vi "Get Parameters And Check Data Types.vi"(8 "error in":errorcluster, 11 "variant":variant) -> (0 "error out":errorcluster, 2 "parameters with invalid type":string[](array[string]), 3 "parameter names":string[](array[string]))   [LabVIEW 2021, in "NI Measurement Plug-In SDK.lvlib"]
uses:
  NI Measurement Plug-In SDK.lvlib
  TypeDefs/Google Protobuf Field Kind.ctl
  <vilib>/Utility/Data Type/NI_Data Type.lvlib
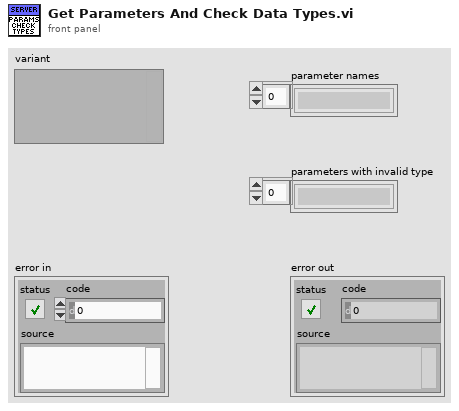
[diagram p1: front panel]
types:
  T1 = typedef "NI Measurement Plug-In SDK.lvlib/Google Protobuf Field Kind.ctl" = enum32{"TYPE_UNKNOWN", "TYPE_DOUBLE", "TYPE_FLOAT", "TYPE_INT64", "TYPE_UINT64", "TYPE_INT32", "TYPE_FIXED64", "TYPE_FIXED32", "TYPE_BOOL", "TYPE_STRING", "TYPE_GROUP", "TYPE_MESSAGE", "TYPE_BYTES", "TYPE_UINT32", "TYPE_ENUM", "TYPE_SFIXED32", "TYPE_SFIXED64", "TYPE_SINT32", "TYPE_SINT64"}
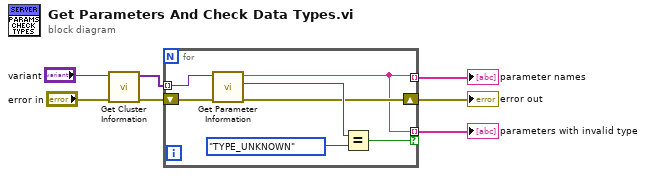
[diagram p0: block diagram]
diagram:
  n1 = call <vilib>:"Get Cluster Information.vi"("error in (no error)"="error in", "variant"="variant") -> ("error out"=w6:errorcluster, "cluster elements"=w5:variant[])  [unwired: 8 in]
  n2 = for {
    tunnel: w5 -> [w14] mode=indexing
    shift-right: [w10] -> w7
    shift-left: w6 -> [w11]
    tunnel: [w8] -> w3 mode=indexing if=w9
    tunnel: [w8] -> w4 mode=indexing
    n3 = call "Get Parameter Information.vi"("error in"=w11, "variant data"=w14) -> ("error out"=w10:errorcluster, "grpc type"=w13:T1, "name"=w8:string)  [unwired: 5 in, 2 out]
    n4 = Equal?(x=w13, y=Google_Protobuf_Field_Kind."TYPE_UNKNOWN") -> (x = y?=w9:bool)
  }
  "parameters with invalid type" <- w3
  "error out" <- w7
  "parameter names" <- w4
